vi "Markers2ColorMap.vi"(11 "Markers-colors":cluster{dbl, u32}[](array[cluster])) -> (3 "ColorMap":u16[](array[numeric]))   [LabVIEW 2018]
uses:
  <vilib>/Analysis/1siggen.llb/Ramp Pattern by Samples.vi
  <vilib>/vision/NI_Vision_Development_Module.lvlib
  <vilib>/Analysis/NI_AALBase.lvlib
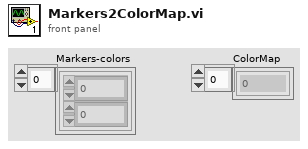
[diagram p1: front panel]
types:
  T1 = cluster{"Red (or Hue) value":u8, "Green (or Sat) value":u8, "Blue (or Light or Val) value":u8}[]
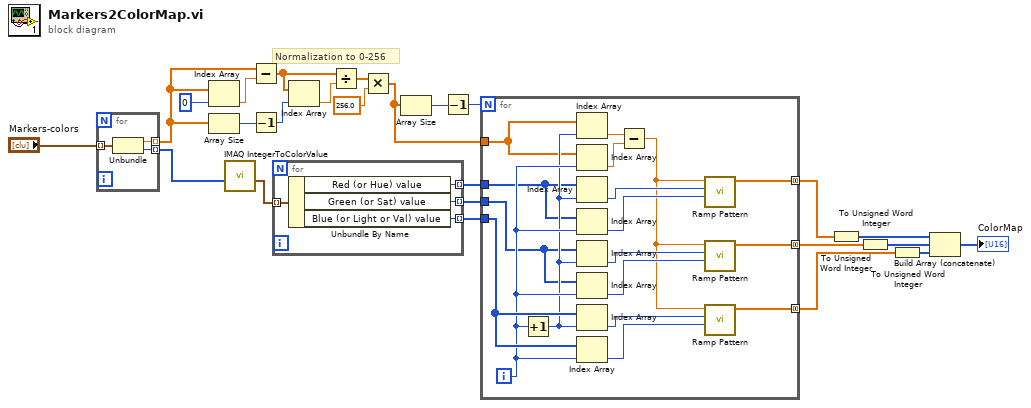
[diagram p0: block diagram]
diagram:
  # "Normalization to 0-256"
  n1 = for {
    tunnel: "Markers-colors" -> [w28] mode=indexing
    tunnel: [w27] -> w9 mode=indexing
    tunnel: [w26] -> w15 mode=indexing
    n2 = Unbundle(w28) -> (w27:dbl, w26:u32)
  }
  n3 = Index Array(array=w9, index=0) -> (element=w12:dbl)
  n4 = Array Size(array=w9) -> (size(s)=w11:i32)
  n5 = call "IMAQ IntegerToColorValue"("1D U32 array"=w15) -> ("1D Color value array"=w16:T1)  [unwired: 4 in, 3 out]
  n6 = Subtract(x=w9, y=w12) -> (x-y=w7:dbl[])
  n7 = Decrement(x=w11) -> (x-1=w10:i32)
  n8 = for {
    tunnel: w16 -> [w32] mode=indexing
    tunnel: [w31] -> w19 mode=indexing
    tunnel: [w30] -> w18 mode=indexing
    tunnel: [w29] -> w17 mode=indexing
    n9 = Unbundle By Name(w32) -> ("Red (or Hue) value"=w31:u8, "Green (or Sat) value"=w30:u8, "Blue (or Light or Val) value"=w29:u8)
  }
  n10 = Index Array(array=w7, index=w10) -> (element=w8:dbl)
  n11 = Divide(x=w7, y=w8) -> (x/y=w5:dbl[])
  n12 = Multiply(x=w5, y=256.0) -> (x*y=w6:dbl[])
  n13 = Array Size(array=w6) -> (size(s)=w20:i32)
  n14 = Decrement(x=w20) -> (x-1=w21:i32)
  n15 = for {
    N: w21 -> [_]
    tunnel: w17 -> [w50]
    tunnel: w18 -> [w40]
    tunnel: w19 -> [w41]
    tunnel: [w36] -> w3 mode=concatenating
    tunnel: [w35] -> w2 mode=concatenating
    tunnel: [w34] -> w1 mode=concatenating
    tunnel: w6 -> [w33]
    i -> [w43]
    n16 = Increment(x=w43) -> (x+1=w42:i32)
    n17 = Index Array(array=w33, index=w42) -> (element=w47:dbl)
    n18 = Index Array(array=w33, index=w43) -> (element=w46:dbl)
    n19 = Index Array(array=w41, index=w42) -> (element=w38:u8)
    n20 = Index Array(array=w41, index=w43) -> (element=w39:u8)
    n21 = Index Array(array=w40, index=w42) -> (element=w44:u8)
    n22 = Index Array(array=w40, index=w43) -> (element=w45:u8)
    n23 = Index Array(array=w50, index=w42) -> (element=w48:u8)
    n24 = Index Array(array=w50, index=w43) -> (element=w49:u8)
    n25 = Subtract(x=w47, y=w46) -> (x-y=w37:dbl)
    n26 = call-poly <vilib>:"Ramp Pattern.vi"("start"=w39, "end"=w38, "samples"=w37) -> ("Ramp Pattern"=w36:dbl[])  [unwired: 7 in, 1 out]
    n27 = call-poly <vilib>:"Ramp Pattern.vi"("start"=w45, "end"=w44, "samples"=w37) -> ("Ramp Pattern"=w35:dbl[])  [unwired: 7 in, 1 out]
    n28 = call-poly <vilib>:"Ramp Pattern.vi"("start"=w49, "end"=w48, "samples"=w37) -> ("Ramp Pattern"=w34:dbl[])  [unwired: 7 in, 1 out]
  }
  n29 = To Unsigned Word Integer(number=w3) -> (unsigned 16bit integer=w23:u16[])
  n30 = To Unsigned Word Integer(number=w2) -> (unsigned 16bit integer=w24:u16[])
  n31 = To Unsigned Word Integer(number=w1) -> (unsigned 16bit integer=w25:u16[])
  n32 = Build Array (concatenate)(w23, w24, w25) -> (→"ColorMap":u16[])
